vi "SetClockSource.vi"(8 "error in (no error)":errorcluster, 10 "Clock Source":u8(ring)=3 items=["Tristate"=0, "Sync Clock (PXIe only)"=2, "Adapter Module Onboard Clock"=3, "Strobe from Crosspoint Switch"=4, "Strobe Bypass"=5], 11 "FPGA VI Reference In":T1) -> (0 "error out":errorcluster, 3 "FPGA VI Reference Out":T1)   [LabVIEW 2012]
uses:
  Common FPGA VIs/Basic_FPGA_Ref.ctl
  <vilib>/Utility/error.llb/Error Cluster From Error Code.vi
  <vilib>/rvi/errors/niLvFpgaAdjustHostInterfaceError.vi
  <vilib>/rvi/interface/nirviReadWriteControl/nirviReadWriteControl.xnode
  <vilib>/rvi/interface/Simulation/niFpgaSimulationCallBeginRW.vi
  NiFpgaLv.dll
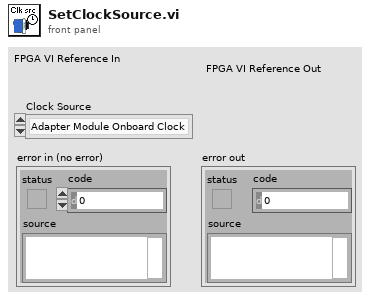
[diagram p1: front panel]
types:
  T1 = typedef "Basic_FPGA_Ref.ctl" = refnum<k20>
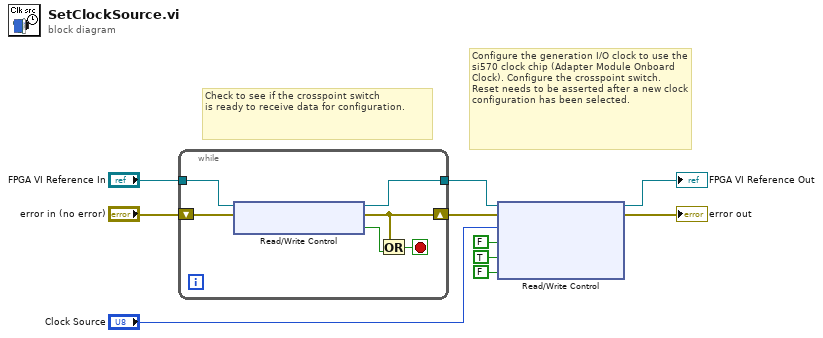
[diagram p0: block diagram]
diagram:
  # "Configure the generation I/O clock to use the si570 clock chip (Adapter Module Onboard Clock). Configure the crosspoint switch. Reset needs to be asserted after a new clock configuration has been selected."
  # "Check to see if the crosspoint switch\nis ready to receive data for configuration."
  n1 = while {
    shift-right: [w14] -> w4
    shift-left: "error in (no error)" -> [w16]
    tunnel: "FPGA VI Reference In" -> [w15]
    tunnel: [w11] -> w5
    stop <- w12 stop-if-true
    n2 = xnode "Read/Write Control"("FPGA VI Reference In"=w15, "error in"=w16) -> ("FPGA VI Reference Out"=w11:T1, "error out"=w14:errorcluster, "Xpoint_Switch_Ready"=w13:bool)
    n3 = Or(x=w14, y=w13) -> (x .or. y?=w12:bool)
  }
  n4 = xnode "Read/Write Control"("FPGA VI Reference In"=w5, "error in"=w4, "Clock Source"="Clock Source", "Xpoint_Switch_Write"=FALSE, "Xpoint_Switch_Write"=TRUE, "Xpoint_Switch_Write"=FALSE) -> ("FPGA VI Reference Out"=→"FPGA VI Reference Out":T1, "error out"=→"error out":errorcluster)
